vi "Load all config.vi"(8 "Error In":errorcluster, 11 "UI data in":T1={"GPIB Addresses"={"GPIB Motor"=2, "GPIB Laser"="3"}, "Beam size"={"BeamX"=1.0, "BeamY"=63.0, "Beam Overlap"=0.0}, "Motor speed"={"Xspeed"=1.0, " Yspeed"=1.0}, "Laser parameters"={"Thyratron Bias"=20.0, "Frequency"=1, "Shots/Point"=1.0}, "Irradiation points"={"X1"=0.0, "Y1"=0.0, "X2"=0.0, "Y2"=0.0}, "Calibration Point"={"Xcalib"=0.0, "Ycalib"=0.0}} {"Laser parameters"."Frequency" format="%.0fHz"; "Laser parameters"."Thyratron Bias" format="%#_gkV"}) -> (0 "Error Out":errorcluster, 3 "UI data out":T1={"GPIB Addresses"={"GPIB Motor"=2, "GPIB Laser"="3"}, "Beam size"={"BeamX"=0.0, "BeamY"=0.0, "Beam Overlap"=0.0}, "Motor speed"={"Xspeed"=0.0, " Yspeed"=0.0}, "Laser parameters"={"Thyratron Bias"=20.0, "Frequency"=0, "Shots/Point"=1.0}, "Irradiation points"={"X1"=0.0, "Y1"=0.0, "X2"=0.0, "Y2"=0.0}, "Calibration Point"={"Xcalib"=-115.0, "Ycalib"=-103.0}} {"Laser parameters"."Frequency" format="%.0fHz"; "Laser parameters"."Thyratron Bias" format="%#_gkV"})   [LabVIEW 2014]
uses:
  Typedef/UI data.ctl
  <vilib>/Utility/config.llb/Read Key (I32).vi
  <vilib>/Utility/config.llb/Read Key (String).vi
  <vilib>/Utility/config.llb/Read Key (Double).vi
  <vilib>/Utility/config.llb/NI_LVConfig.lvlib
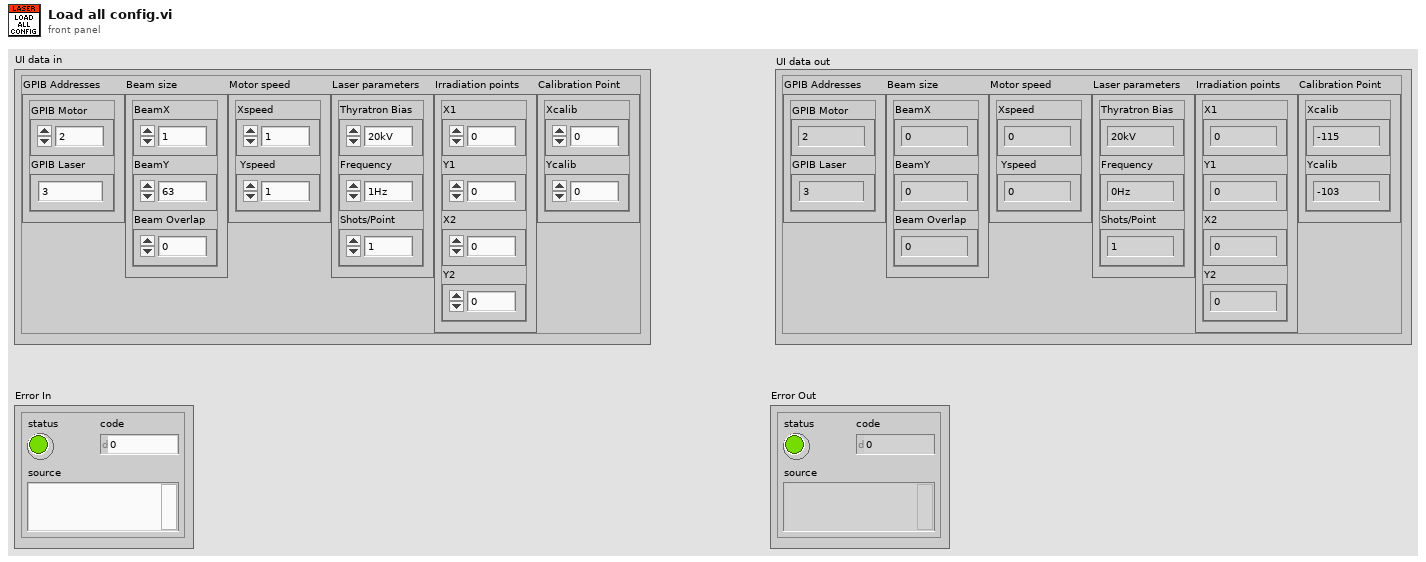
[diagram p1: front panel]
types:
  T1 = typedef "UI data.ctl" = cluster{"GPIB Addresses":cluster{"GPIB Motor":i16, "GPIB Laser":string}, "Beam size":cluster{"BeamX":dbl, "BeamY":dbl, "Beam Overlap":dbl}, "Motor speed":cluster{"Xspeed":dbl, " Yspeed":dbl}, "Laser parameters":cluster{"Thyratron Bias":dbl, "Frequency":u16, "Shots/Point":dbl}, "Irradiation points":cluster{"X1":dbl, "Y1":dbl, "X2":dbl, "Y2":dbl}, "Calibration Point":cluster{"Xcalib":dbl, "Ycalib":dbl}}
  T2 = typedef "NI_LVConfig.lvlib/Config Data RefNum.ctl" = refnum<k1>
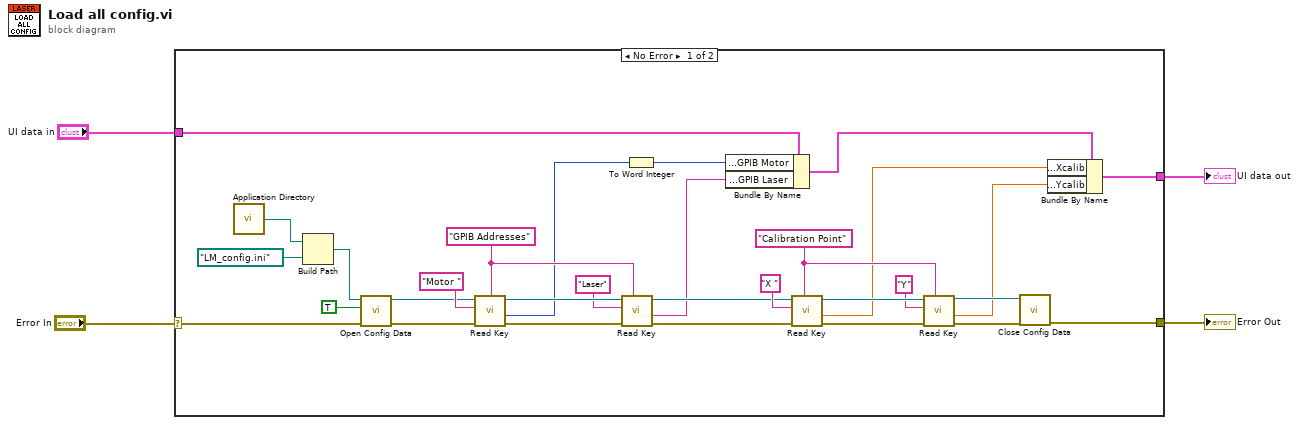
[diagram p0: block diagram]
diagram:
  n1 = case shown="No Error" "Error In" {
    selector: "Error In" -> [w34 w36]
    tunnel: "UI data in" -> [w9 w35]
    tunnel: [w20 w35] -> w2
    tunnel: [w19 w36] -> w1
    frame No Error {
      w18 = "GPIB Addresses" ("section")
      w29 = "Calibration Point" ("section")
      n2 = call <vilib>:"Application Directory.vi"() -> ("Application Directory"=w33:path)
      n3 = Build Path(base path=w33, name or relative path=path "LM_config.ini" ("default name")) -> (appended path=w31:path)
      n4 = call <vilib>:"Open Config Data.vi"("error in (no error)"=w34, "create file if necessary (T)"=TRUE, "configuration file path"=w31) -> ("error out"=w13:errorcluster, "refnum"=w12:T2)  [unwired: 6 in, 1 out]
      n5 = call-poly <vilib>:"Read Key.vi"("section"=w18, "error in (no error)"=w13, "key"="Motor ", "refnum"=w12) -> ("error out"=w17:errorcluster, "value"=w6:i32, "refnum out"=w16:T2)  [unwired: 4 in, 1 out]
      n6 = call-poly <vilib>:"Read Key.vi"("section"=w18, "error in (no error)"=w17, "key"="Laser", "refnum"=w16) -> ("error out"=w10:errorcluster, "value"=w5:string, "refnum out"=w11:T2)  [unwired: 4 in, 1 out]
      n7 = To Word Integer(number=w6) -> (16bit integer=w7:i16)
      n8 = Bundle By Name(cluster=w9, "GPIB Addresses.GPIB Motor"=w7, "GPIB Addresses.GPIB Laser"=w5) -> (w8:T1)
      n9 = call-poly <vilib>:"Read Key.vi"("section"=w29, "error in (no error)"=w10, "key"="X ", "refnum"=w11) -> ("error out"=w28:errorcluster, "value"=w22:dbl, "refnum out"=w27:T2)  [unwired: 4 in, 1 out]
      n10 = call-poly <vilib>:"Read Key.vi"("section"=w29, "error in (no error)"=w28, "key"="Y", "refnum"=w27) -> ("error out"=w24:errorcluster, "value"=w21:dbl, "refnum out"=w23:T2)  [unwired: 4 in, 1 out]
      n11 = call <vilib>:"Close Config Data.vi"("error in (no error)"=w24, "refnum"=w23) -> ("error out"=w19:errorcluster)  [unwired: 8 in, 1 out]
      n12 = Bundle By Name(cluster=w8, "Calibration Point.Xcalib"=w22, "Calibration Point.Ycalib"=w21) -> (w20:T1)
    }
    frame Error {
    }
  }
  "Error Out" <- w1
  "UI data out" <- w2
